vi "CLSUIP_MemberTemplate.vi"(8 "error in":errorcluster, 11 "DNL_LabVIEW Object in":refnum<class>) -> (0 "error out":errorcluster, 3 "DNL_LabVIEW Object out":refnum<class>)   [LabVIEW 2024]
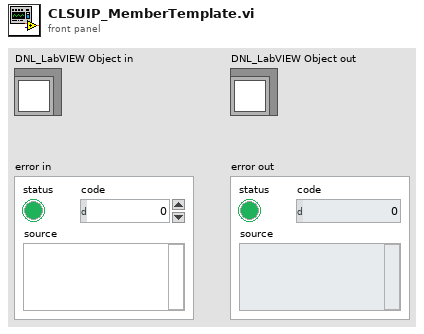
[diagram p1: front panel]
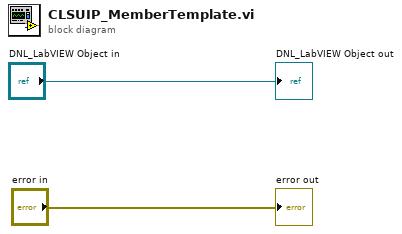
[diagram p0: block diagram]
diagram:
  "DNL_LabVIEW Object out" <- "DNL_LabVIEW Object in"
  "error out" <- "error in"
